vi "modal_hit.vi"(8 "error in":errorcluster, 11 "data_in":T1 {"config"."updateTime" format="%#_g ms"; "config"."lowPass" format="%#_g Hz"; "config"."highPass" format="%#_g Hz"; "config"."cutoff" format="%#_g dB"; "config"."preTrigger" format="%#_g ms"; "config"."thr" format="%#_g N"; "config"."duration" format="%#_g s"; "config"."rate" min=1652.0 max=51200.0 format="%#_g Hz"}) -> (0 "error out":errorcluster, 3 "data_out":T1 {"config"."updateTime" format="%#_g ms"; "config"."lowPass" format="%#_g Hz"; "config"."highPass" format="%#_g Hz"; "config"."cutoff" format="%#_g dB"; "config"."preTrigger" format="%#_g ms"; "config"."thr" format="%#_g N"; "config"."duration" format="%#_g s"; "config"."rate" min=1652.0 max=51200.0 format="%#_g Hz"})   [LabVIEW 2016]
uses:
  results_data.ctl
  MainFGV/Settings/Advanced/AdvancedConfig.ctl
  <vilib>/Analysis/NI_AALPro.lvlib
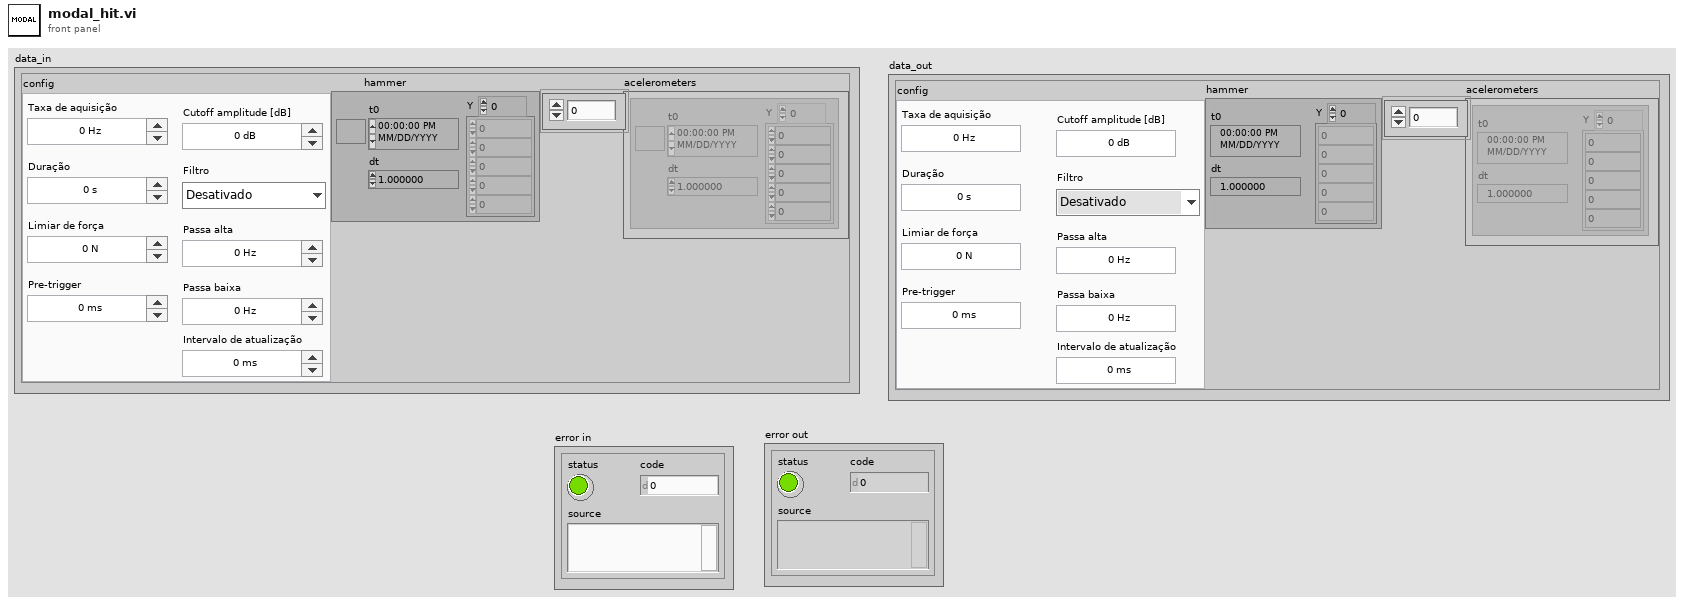
[diagram p1: front panel]
types:
  T1 = typedef "results_data.ctl" = cluster{"config":T2, "hammer":waveform(dbl), "acelerometers":waveform(dbl)[]}
  T2 = typedef "AdvancedConfig.ctl" = cluster{"rate":dbl, "duration":dbl, "thr":dbl, "preTrigger":dbl, "cutoff":dbl, "Filtro":enum16{"Desativado", "Passa banda", "Passa alta", "Passa baixa"}, "highPass":dbl, "lowPass":dbl, "updateTime":dbl}
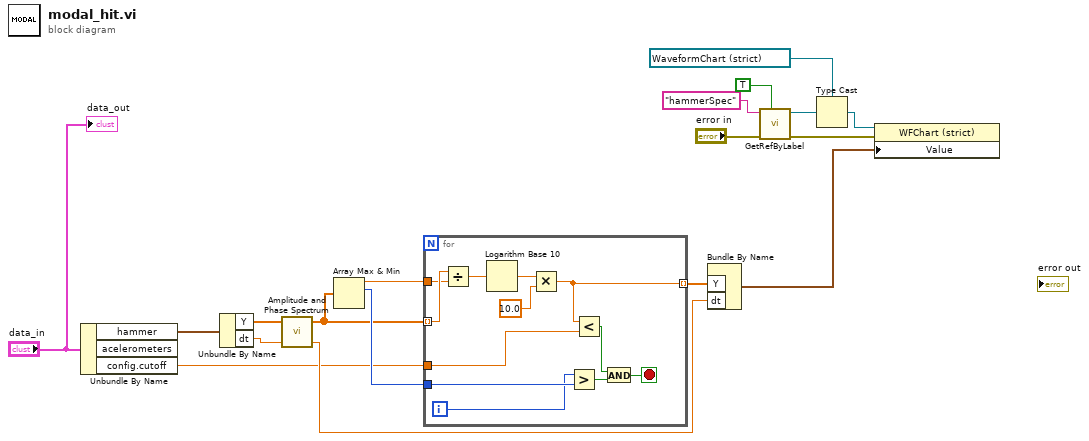
[diagram p0: block diagram]
diagram:
  n1 = Unbundle By Name("data_in") -> ("hammer"=w17:waveform(dbl), "config.cutoff"=w2:dbl)  [unwired: 1 out]
  n2 = Unbundle By Name(w17) -> ("Y"=w16:dbl[], "dt"=w15:dbl)
  n3 = call <vilib>:"Amplitude and Phase Spectrum.vi"("dt"=w15, "Signal (V)"=w16) -> ("df"=w12:dbl, "Amp Spectrum Mag (Vrms)"=w13:dbl[])  [unwired: 1 in, 1 out]
  n4 = Array Max & Min(array=w13) -> (max value=w3:dbl, max index (indices)=w14:i32)  [unwired: 2 out]
  n5 = for {
    tunnel: w13 -> [w25] mode=indexing
    tunnel: w14 -> [w30]
    tunnel: w3 -> [w24]
    tunnel: w2 -> [w20]
    tunnel: [w19] -> w1 mode=indexing
    i -> [w26]
    stop <- w27 stop-if-true
    n6 = Divide(x=w25, y=w24) -> (x/y=w23:dbl)
    n7 = Logarithm Base 10(1:w23) -> (0:w22:dbl)
    n8 = Multiply(x=w22, y=10.0) -> (x*y=w19:dbl)
    n9 = Greater?(x=w26, y=w30) -> (0:w29:bool)
    n10 = Less?(x=w19, y=w20) -> (x < y?=w28:bool)
    n11 = And(x=w28, y=w29) -> (x .and. y?=w27:bool)
  }
  n12 = Bundle By Name("Y"=w1, "dt"=w12) -> (w4:waveform(dbl))  [unwired: 1 in]
  n13 = call "GetRefByLabel.vi"("InsideTab"=TRUE, "error in"="error in", "Label"="hammerSpec") -> ("error out"=w6:errorcluster, "Ctl Refnum"=w7:refnum<vi>)  [unwired: 6 in, 1 out]
  n14 = Type Cast(type=refnum<vi> refnum ("hammerTime"), x=w7) -> (*(type *) &x=w5:refnum<vi>)
  n15 = property class="WFChart (strict)"(reference=w5, error in=w6, "Value"=w4) -> ()  [unwired: 2 out]
  "data_out" <- "data_in"
